vi "INST_PS_SET_CURR_LIMIT_1.0.0.vi"(4 "Use OPC(T)":bool, 6 "Instrument Select (Output 1)":string(combo)="OUT1", 8 "error in (no error)":errorcluster, 9 "Curr Limit (A)":dbl, 10 "Curr Limit (A)str":string, 11 "VISA session":refnum<visa-resource-name>) -> (0 "error out":errorcluster, 3 "dup VISA session":refnum<visa-resource-name>)   [LabVIEW 2018]
doc: "This VI configures the DC voltage level the power supply attempts to generate."
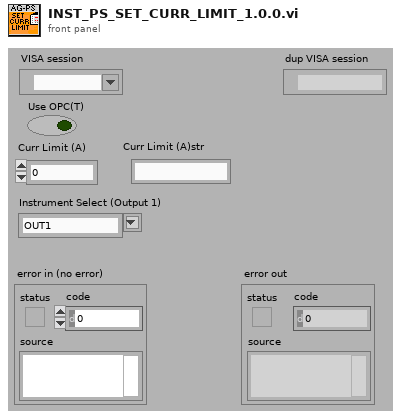
[diagram p1: front panel]
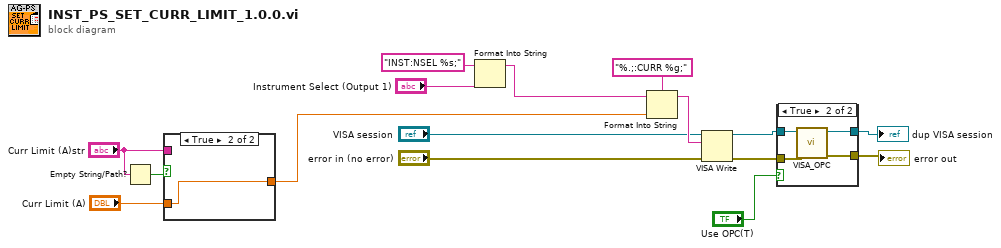
[diagram p0: block diagram]
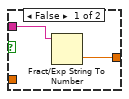
[diagram p2: hidden frame]
diagram:
  n1 = Empty String/Path?(string/path="Curr Limit (A)str") -> (empty?=w7:bool)
  n2 = case shown="True" w7 {
    tunnel: "Curr Limit (A)str" -> [w18 _]
    tunnel: [w17 w19] -> w5
    tunnel: "Curr Limit (A)" -> [_ w19]
    frame False {
      n3 = Fract/Exp String To Number(string=w18) -> (number=w17:dbl)  [unwired: 3 in, 1 out]
    }
    frame True {
    }
  }
  n4 = Format Into String(format string="INST:NSEL %s;", "Instrument Select (Output 1)") -> (resulting string=w3:string)  [unwired: 2 in, 1 out]
  n5 = Format Into String(format string="%.;:CURR %g;", initial string=w3, w5) -> (resulting string=w15:string)  [unwired: 1 in, 1 out]
  n6 = VISA Write(VISA resource name="VISA session", write buffer=w15, error in (no error)="error in (no error)") -> (VISA resource name out=w9:refnum<visa-resource-name>, error out=w16:errorcluster)  [unwired: 1 out]
  n7 = case shown="True" "Use OPC(T)" {
    tunnel: w16 -> [w21 w25]
    tunnel: [w21 w24] -> w11
    tunnel: w9 -> [w20 w23]
    tunnel: [w20 w22] -> w8
    frame False {
    }
    frame True {
      n8 = call "VISA_OPC.vi"("error in"=w25, "Session In"=w23) -> ("error out"=w24:errorcluster, "Session Out"=w22:refnum<visa-resource-name>)  [unwired: 7 in, 1 out]
    }
  }
  "error out" <- w11
  "dup VISA session" <- w8
